vi "CreateHTTPResponse.vi"(10 "Http Response Codes":T1=403 items=["Forbidden"=403, "Not Found"=404, "Upgrade Required"=426]) -> (2 "Http Response":string)   [LabVIEW 2021, in "LV WebSockets.lvlib"]
uses:
  LV WebSockets.lvlib
  HTTPResponseCodes.ctl
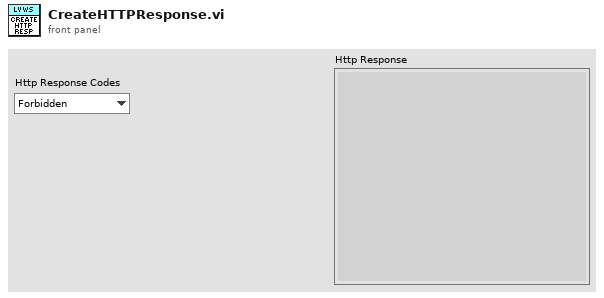
[diagram p1: front panel]
types:
  T1 = typedef "LV WebSockets.lvlib/HTTPResponseCodes.ctl" = u16
  T2 = typedef "LVStringsAndValuesArrayTypeDef_U16.ctl" = cluster{"String":string, "Value":u16}[]
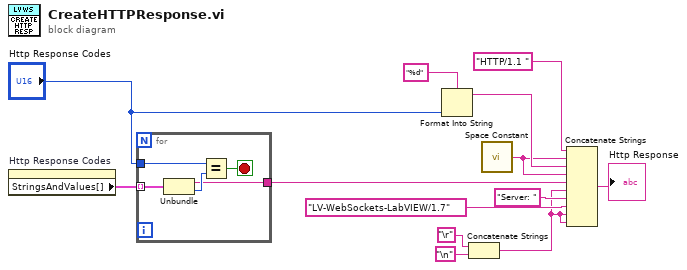
[diagram p0: block diagram]
diagram:
  n1 = property on="Http Response Codes" class="Ring (strict)"() -> ("StringsAndValues[]"=w8:T2)  [unwired: 2 in, 2 out]
  n2 = for {
    tunnel: w8 -> [w18] mode=indexing
    tunnel: "Http Response Codes" -> [w16]
    tunnel: [w14] -> w6
    stop <- w15 stop-if-true
    n3 = Unbundle(w18) -> ("String"=w14:string, "Value"=w17:u16)
    n4 = Equal?(x=w16, y=w17) -> (x = y?=w15:bool)
  }
  n5 = Format Into String(format string="%d", "Http Response Codes") -> (resulting string=w11:string)  [unwired: 2 in, 1 out]
  n6 = Concatenate Strings("\r", "\n") -> (w1:string)
  n7 = call <vilib>:"Space Constant.vi"() -> ("String"=w10:string)
  n8 = Concatenate Strings("HTTP/1.1 ", w10, w11, w10, w6, w1, "Server: " ("string"), "LV-WebSockets-LabVIEW/1.7" ("string"), w1, w1) -> (→"Http Response":string)
